vi "File Save.vi"(8 "error in (no error)":errorcluster, 11 "LF2R IDE in":refnum<class "LF2R IDE.lvclass">) -> (0 "error out":errorcluster, 1 "File Exist?":bool, 3 "LF2R IDE out":refnum<class "LF2R IDE.lvclass">)   [LabVIEW 2018, in "LF2R IDE.lvlib" / "LF2R IDE.lvclass"]
uses:
  LF2R IDE.lvclass
  LF2R IDE.lvclass/LF2R IDE.ctl
  ScintillaNET/ScintillaNET.lvclass
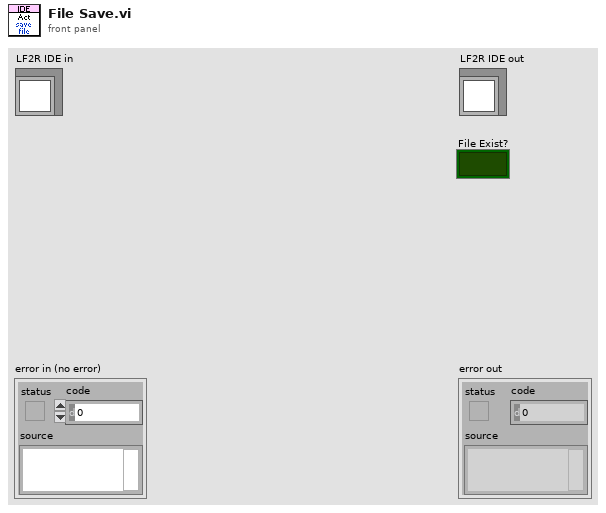
[diagram p1: front panel]
types:
  T1 = enum16{"open", "replace", "create", "open or create", "replace or create", "replace or create with confirmation"}
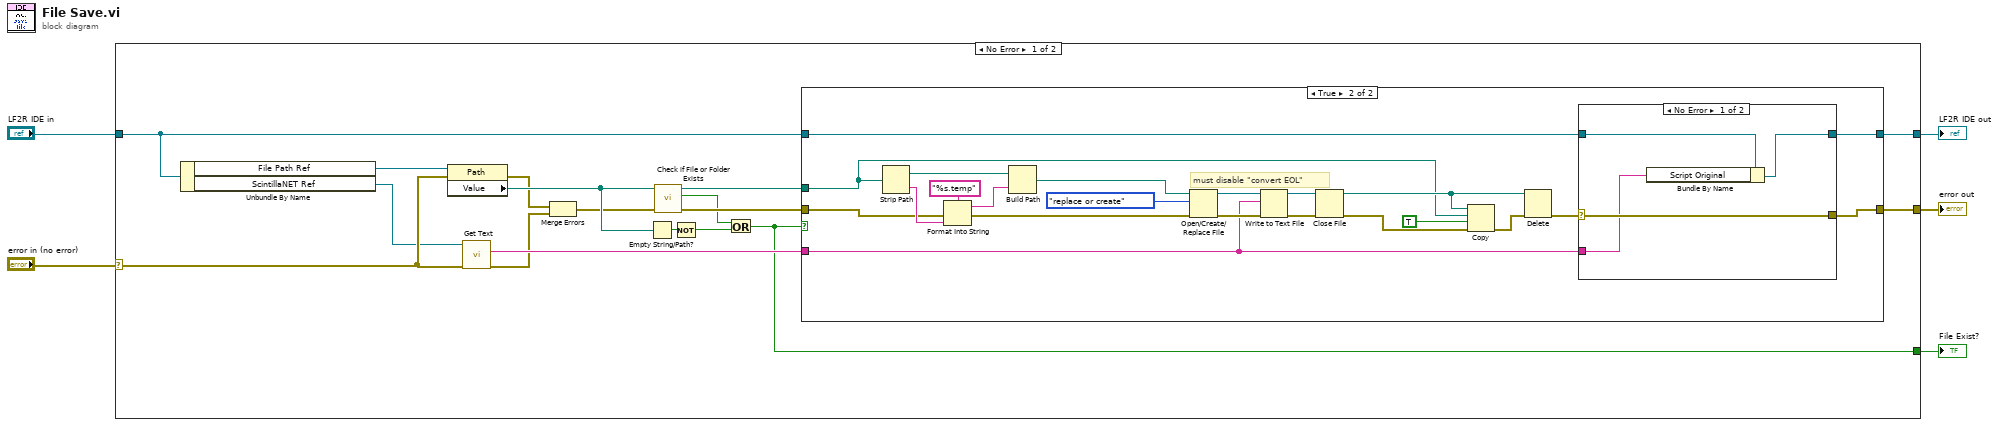
[diagram p0: block diagram]
diagram:
  n1 = case shown="No Error" "error in (no error)" {
    selector: "error in (no error)" -> [w11 w54]
    tunnel: [w13 w54] -> w4
    tunnel: [w19 w53] -> w2
    tunnel: "LF2R IDE in" -> [w20 w53]
    tunnel: [w6 _] -> w1
    frame No Error {
      n2 = Unbundle By Name(w20) -> ("File Path Ref"=w22:refnum<vi>, "ScintillaNET Ref"=w10:refnum<class "ScintillaNET.lvclass">)
      n3 = property class="Path"(reference=w22, error in=w11) -> (error out=w8:errorcluster, "Value"=w18:path)  [unwired: 1 out]
      n4 = call "Get Text.vi"("error in (no error)"=w11, "ScintillaNET in"=w10) -> ("error out"=w9:errorcluster, "Text"=w12:string)  [unwired: 7 in, 1 out]
      n5 = Merge Errors(w8, w9) -> (w7:errorcluster)
      n6 = Empty String/Path?(string/path=w18) -> (empty?=w21:bool)
      n7 = call <vilib>:"Check if File or Folder Exists.vi"("error in (no error)"=w7, "path"=w18) -> ("error out"=w16:errorcluster, "file or folder exists?"=w15:bool, "dup path"=w17:path)  [unwired: 7 in]
      n8 = Not(x=w21) -> (.not. x?=w14:bool)
      n9 = Or(x=w15, y=w14) -> (x .or. y?=w6:bool)
      n10 = case shown="True" w6 {
        tunnel: w20 -> [w24 w29]
        tunnel: [w24 w28] -> w19
        tunnel: w17 -> [_ w31]
        tunnel: w16 -> [w23 w30]
        tunnel: w12 -> [_ w25]
        tunnel: [w23 w26] -> w13
        frame False {
        }
        frame True {
          # "must disable \"convert EOL\""
          n11 = Strip Path(path=w31) -> (stripped path=w42:path, name=w41:string)
          n12 = Format Into String(format string="%s.temp", error in=w30, w41) -> (resulting string=w39:string, error out=w37:errorcluster)  [unwired: 1 in]
          n13 = Build Path(base path=w42, name or relative path=w39) -> (appended path=w38:path)
          n14 = Open/Create/Replace File(file path (use dialog)=w38, error in=w37, operation (0:open)=T1."replace or create") -> (refnum out=w46:refnum<file>, error out=w45:errorcluster)  [unwired: 3 in, 1 out]
          n15 = Write to Text File(file (use dialog)=w46, text=w25, error in=w45) -> (refnum out=w44:refnum<file>, error out=w43:errorcluster)  [unwired: 1 in, 1 out]
          n16 = Close File(refnum=w44, error in=w43) -> (path=w32:path, error out=w36:errorcluster)
          n17 = Copy(8:w36, 9:TRUE ("overwrite (F)"), 10:w31, 11:w32) -> (0:w34:errorcluster)  [unwired: 1 in, 2 out]
          n18 = Delete(path (use dialog)=w32, error in=w34) -> (error out=w27:errorcluster)  [unwired: 3 in, 2 out]
          n19 = case shown="No Error" w27 {
            selector: w27 -> [w48 w51]
            tunnel: w29 -> [w50 w52]
            tunnel: [w49 w52] -> w28
            tunnel: [w48 w51] -> w26
            tunnel: w25 -> [w47 _]
            frame No Error {
              n20 = Bundle By Name(cluster=w50, "Script Original"=w47) -> (w49:refnum<class "LF2R IDE.lvclass">)
            }
            frame Error {
            }
          }
        }
      }
    }
    frame Error {
    }
  }
  "error out" <- w4
  "LF2R IDE out" <- w2
  "File Exist?" <- w1
